vi "Read State.vi"(8 "error in (no error)":errorcluster, 11 "Measure Object in":refnum<class "Worker.lvclass">) -> (0 "error out":errorcluster, 2 "State":T1, 3 "Measure Object out":refnum<class "Worker.lvclass">)   [LabVIEW 2016, in "Worker.lvclass"]
uses:
  Worker/Worker.lvclass
  Worker/Worker State.ctl
  Worker/Worker.lvclass/Worker.ctl
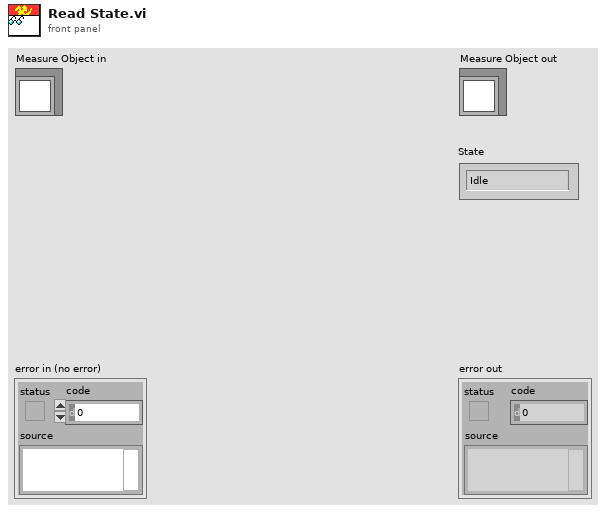
[diagram p1: front panel]
types:
  T1 = typedef "Worker State.ctl" = enum16{"Idle", "Starting", "Working", "Stopping"}
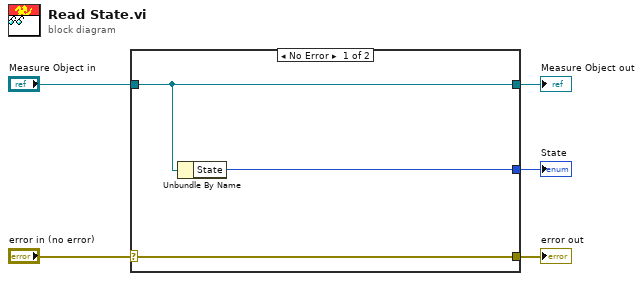
[diagram p0: block diagram]
diagram:
  n1 = case shown="No Error" "error in (no error)" {
    selector: "error in (no error)" -> [w8 w9]
    tunnel: [w8 w9] -> w4
    tunnel: [w7 w10] -> w2
    tunnel: "Measure Object in" -> [w7 w10]
    tunnel: [w6 _] -> w1
    frame No Error {
      n2 = Unbundle By Name(w7) -> ("State"=w6:T1)
    }
    frame Error {
    }
  }
  "error out" <- w4
  "Measure Object out" <- w2
  "State" <- w1
